vi "Check_Traverse_move.vi"(0 "Current position":dbl[](array[numeric])=[0.0, 0.0, 0.0] format="%.2f", 1 "Traverse Name":string, 2 "Full Check":bool, 5 "New Position":dbl[](array[numeric])=[0.0, 0.0, 0.0] format="%.2f", 7 "Model       Roll      Pitch       Yaw (deg)":dbl[](array[numeric]) format="%#.2f", 9 "Probe Volume":T1=[{"Max"=15.0, "Min"=-15.0}, {"Max"=250.0, "Min"=0.0}, {"Max"=15.0, "Min"=-15.0}] {"Min" format="%#.1f"; "Max" format="%#.1f"}, 11 "Entire Space":T1=[{"Max"=15001.0, "Min"=12000.0}, {"Max"=1000.0, "Min"=-1000.0}, {"Max"=700.0, "Min"=0.0}] {"Min" format="%#.1f"; "Max" format="%#.1f"}, 12 "Exclude Array":T2[](array[typedef])=[{"Sizes"=[{"Max"=15000.0, "Min"=0.0}, {"Max"=1000.0, "Min"=-1000.0}, {"Max"=300.0, "Min"=0.0}], "Name"="Roughness Elements", "Exclude Type"=enum."Allow only vertical moves"}, {"Sizes"=[{"Max"=17000.0, "Min"=16000.0}, {"Max"=200.0, "Min"=-200.0}, {"Max"=-50.0, "Min"=-250.0}], "Name"="B204", "Exclude Type"=enum."Exclude completely"}] {"Sizes"."Min" format="%#.1f"; "Sizes"."Max" format="%#.1f"}, 13 "Probe Support":T1=[{"Max"=15001.0, "Min"=12000.0}, {"Max"=1000.0, "Min"=-1000.0}, {"Max"=700.0, "Min"=0.0}] {"Min" format="%#.1f"; "Max" format="%#.1f"}) -> (6 "Position At Crash":dbl[](array[numeric]) format="%.2f", 10 "Steps":dbl[][](array[numeric]) format="%.2f", 15 "Error Comments":string)   [LabVIEW 2013]
uses:
  Box_size.ctl
  Exclude_cluster.ctl
  Exclusion_type.ctl
panel:
  # "X                Y                   Z"
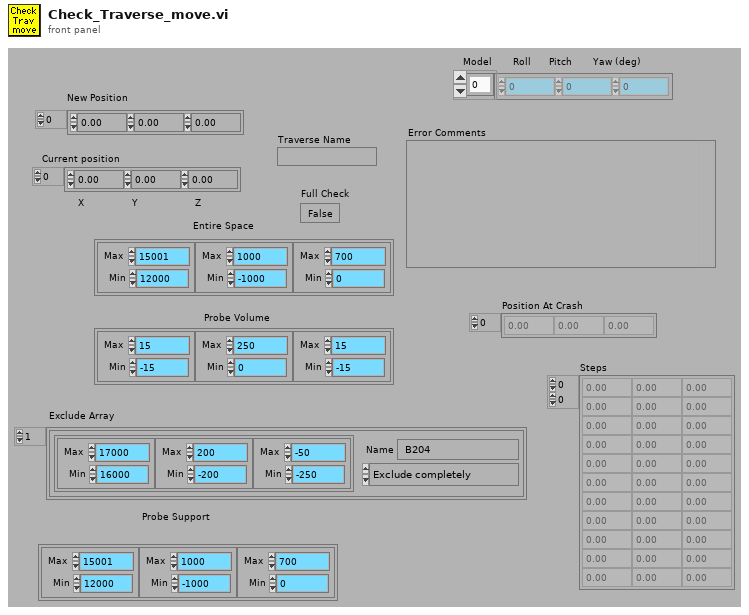
[diagram p1: front panel]
types:
  T1 = typedef "Box_size.ctl" = cluster{"Max":dbl, "Min":dbl}[]
  T2 = typedef "Exclude_cluster.ctl" = cluster{"Sizes":T1, "Name":string, "Exclude Type":T3}
  T3 = typedef "Exclusion_type.ctl" = enum16{"Exclude completely", "Allow only vertical moves"}
  T4 = enum16{"To Traverse Coordinates", "To User Coordinates"}
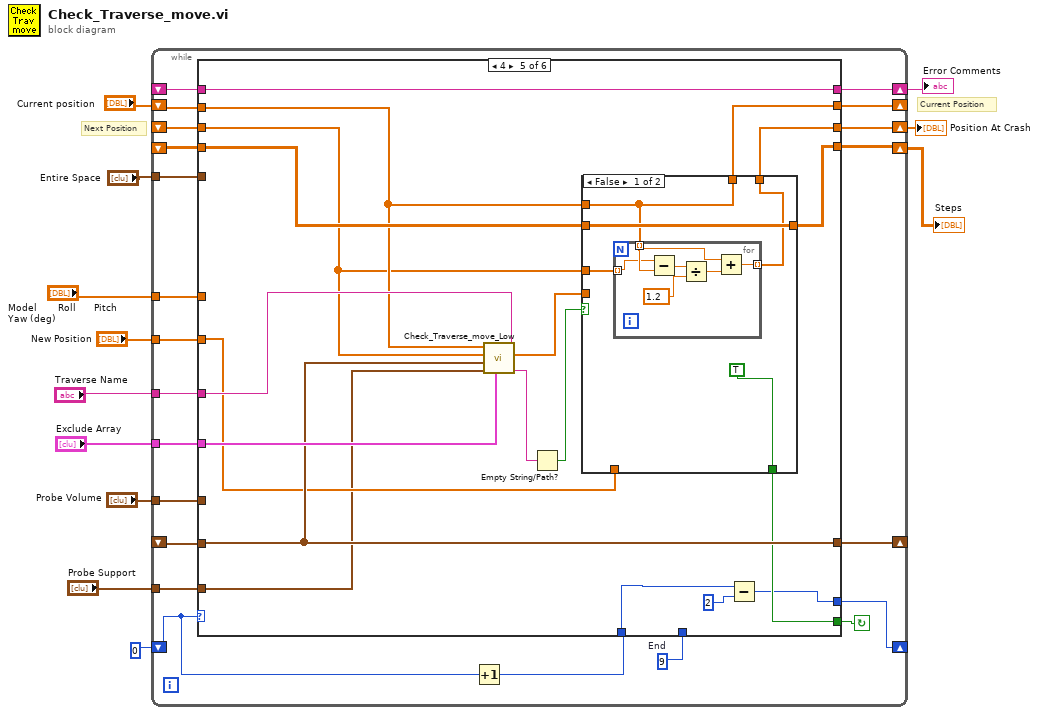
[diagram p0: block diagram]
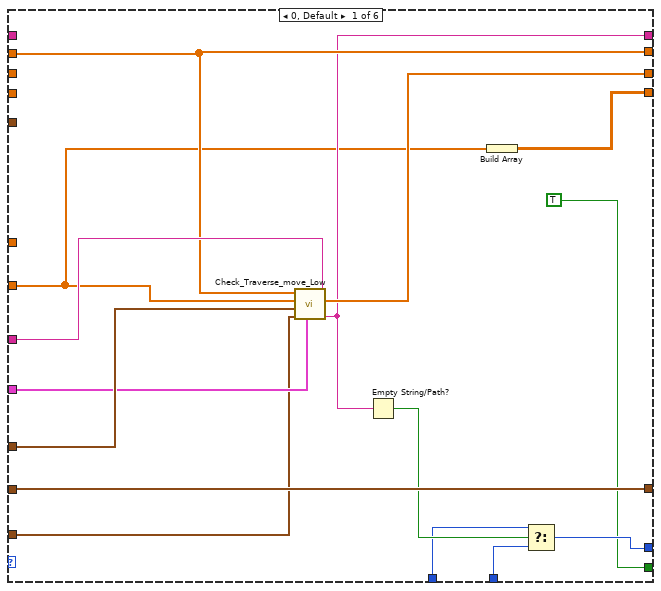
[diagram p2: hidden frame]
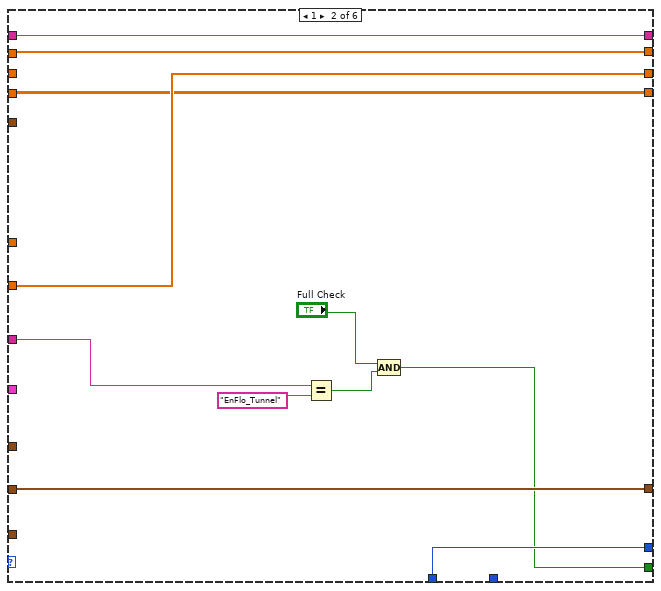
[diagram p3: hidden frame]
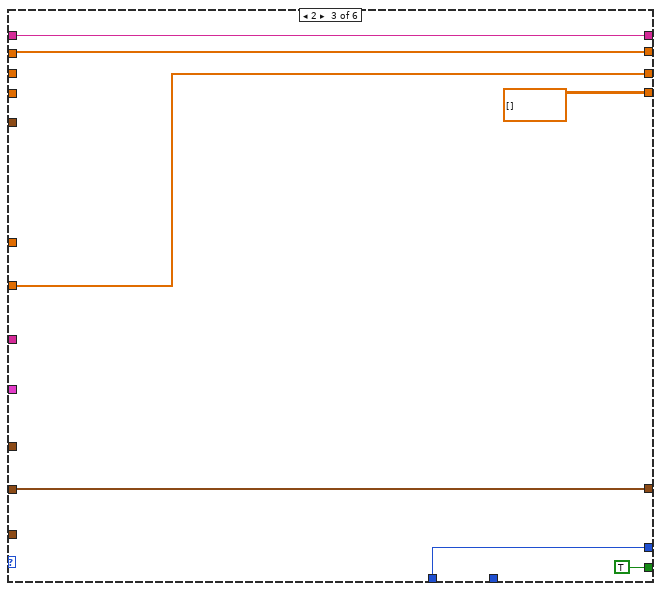
[diagram p4: hidden frame]
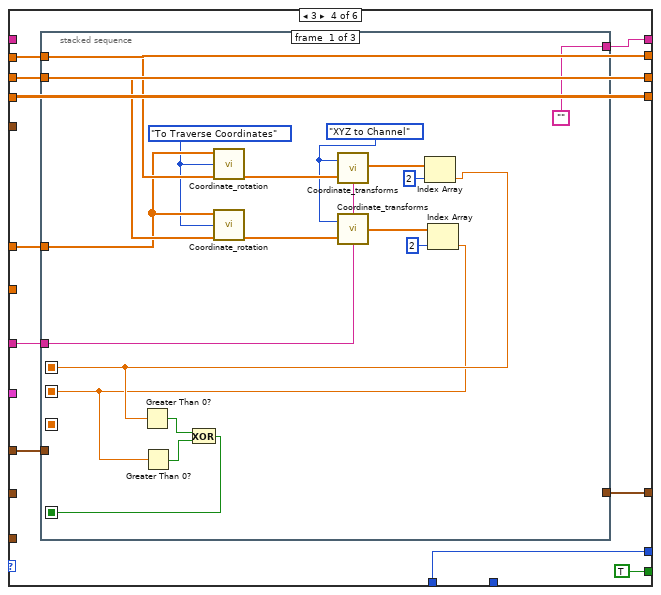
[diagram p5: hidden frame]
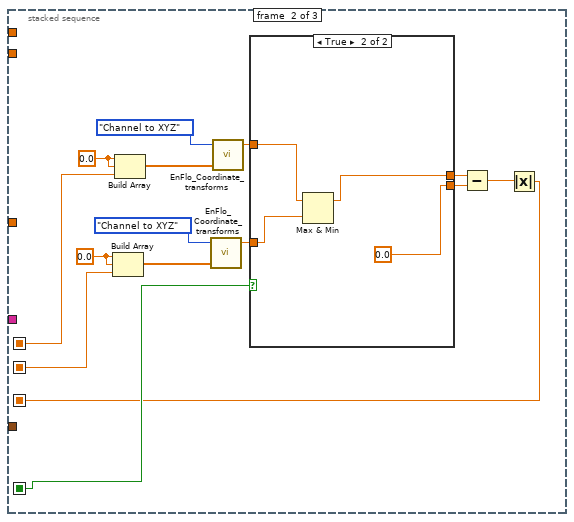
[diagram p6: hidden frame]
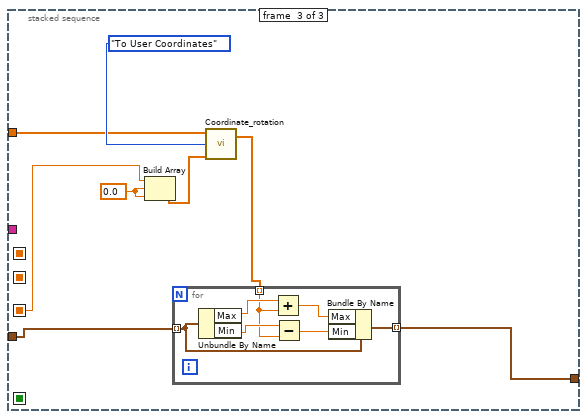
[diagram p8: hidden frame]
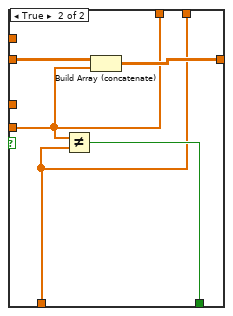
[diagram p9: hidden frame]
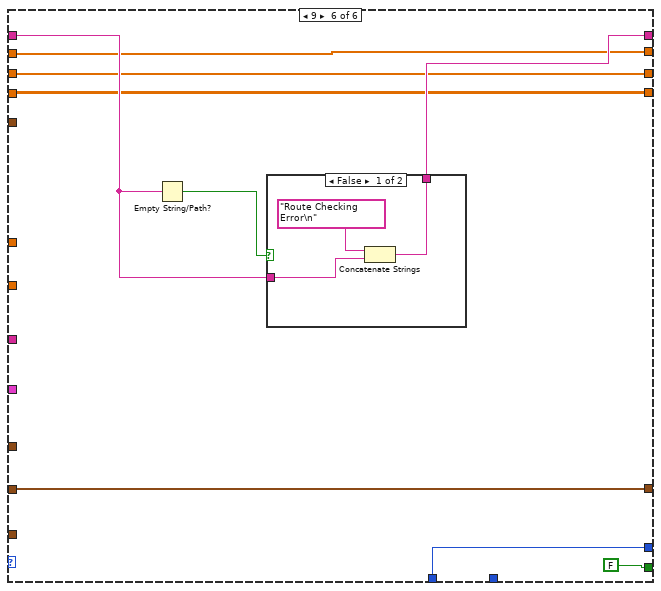
[diagram p10: hidden frame]
diagram:
  # "Current Position"
  # "Next Position"
  n1 = while {
    shift-left: _ -> [w15]
    shift-right: [w14] -> w3
    tunnel: "Probe Volume" -> [w17]
    shift-left: _ -> [w19]
    shift-right: [w18] -> _
    tunnel: "Model       Roll      Pitch       Yaw (deg)" -> [w20]
    tunnel: "New Position" -> [w21]
    shift-left: _ -> [w23]
    shift-right: [w24] -> w7
    shift-left: 0 -> [w27]
    shift-right: [w26] -> _
    tunnel: "Traverse Name" -> [w28]
    tunnel: "Entire Space" -> [w29]
    tunnel: "Exclude Array" -> [w30]
    shift-left: _ -> [w22]
    shift-right: [w32] -> w5
    shift-left: "Current position" -> [w34]
    shift-right: [w33] -> _
    tunnel: "Probe Support" -> [w13]
    stop <- w31 continue-if-true
    w16 = 9  # End
    n2 = Increment(x=w27) -> (x+1=w25:i32)
    n3 = case shown="4" w27 {
      tunnel: w34 -> [w44 w59 w66 w74 w134 w169]
      tunnel: [w44 w59 w66 w74 w139 w169] -> w33
      tunnel: [w47 w52 w63 w73 w138 w168] -> w32
      tunnel: [TRUE ("Box Inside") w54 TRUE ("Box Inside") TRUE ("Box Inside") w141 FALSE ("Box Inside")] -> w31
      tunnel: w19 -> [w46 w58 w65 _ w148 w170]
      tunnel: w30 -> [w48 _ _ _ w150 _]
      tunnel: w29 -> [_ _ _ _ _ _]
      tunnel: w28 -> [w45 w55 _ w71 w149 _]
      tunnel: [w39 w57 w64 w69 w136 w172] -> w26
      tunnel: w25 -> [w41 w57 w64 w69 w135 w172]
      tunnel: [w43 w60 w67 w77 w146 w173] -> w24
      tunnel: w23 -> [_ w60 w67 _ w146 w174]
      tunnel: w22 -> [_ _ _ w73 w133 w168]
      tunnel: w21 -> [w38 w52 w63 _ w142 _]
      tunnel: w20 -> [_ _ _ w72 _ _]
      tunnel: [w46 w58 w65 w75 w148 w170] -> w18
      tunnel: w17 -> [w49 _ _ w70 _ _]
      tunnel: w16 -> [w40 _ _ _ _ _]
      tunnel: w15 -> [_ w51 _ w68 w145 w167]
      tunnel: [w37 w51 dbl[][] [] w68 w144 w167] -> w14
      tunnel: w13 -> [w35 _ _ _ w132 _]
      frame 0, Default {
        n4 = call "Check_Traverse_move_Low.vi"("Traverse Name"=w45, "Exclude Array"=w48, "Probe Support"=w35, "Probe Volume"=w49, "New Position"=w38, "Current position"=w44) -> ("Error Comments"=w43:string, "Position At Crash"=w47:dbl[])  [unwired: 1 in, 1 out]
        n5 = Empty String/Path?(string/path=w43) -> (empty?=w42:bool)
        n6 = Build Array(w38) -> (w37:dbl[][])
        n7 = Select(t=w41, s=w42, f=w40) -> (s? t:f=w39:i32)
      }
      frame 1 {
        n8 = Equal?(x=w55, y="EnFlo_Tunnel") -> (x = y?=w50:bool)
        n9 = Compound Arithmetic op=AND("Full Check", w50) -> (w54:bool)
      }
      frame 2 {
      }
      frame 3 {
        n10 = stacked-sequence {
          seq-local: [w80 _ _] -> [_ w110 _]
          seq-local: [w79 _ _] -> [_ w109 _]
          seq-local: [w78 _ _] -> [_ w100 _]
          seq-local: [_ w96 _] -> [_ _ w119]
          tunnel: ["" _ _] -> w77
          tunnel: [_ _ w123] -> w75
          tunnel: w74 -> [w93 _ _]
          tunnel: w73 -> [w91 _ _]
          tunnel: w72 -> [w90 _ w117]
          tunnel: w71 -> [w89 _ _]
          tunnel: w70 -> [_ _ w124]
          frame #0 {
            w87 = enum16{"XYZ to Channel", "Channel to XYZ"}."XYZ to Channel" ("Mode")
            w88 = T4."To Traverse Coordinates" ("Mode")
            n11 = call "Coordinate_rotation.vi"("Model       Roll      Pitch       Yaw (deg)"=w90, "Input Position"=w93, "Mode"=w88) -> ("Output Position"=w94:dbl[])  [unwired: 2 in, 1 out]
            n12 = call "Coordinate_rotation.vi"("Model       Roll      Pitch       Yaw (deg)"=w90, "Input Position"=w91, "Mode"=w88) -> ("Output Position"=w92:dbl[])  [unwired: 2 in, 1 out]
            n13 = call "Coordinate_transforms.vi"("Traverse Name"=w89, "Input"=w94, "Mode"=w87) -> ("Output"=w86:dbl[])
            n14 = call "Coordinate_transforms.vi"("Traverse Name"=w89, "Input"=w92, "Mode"=w87) -> ("Output"=w83:dbl[])
            n15 = Index Array(array=w86, index=2) -> (element=w80:dbl)
            n16 = Greater Than 0?(x=w80) -> (x > 0?=w82:bool)
            n17 = Index Array(array=w83, index=2) -> (element=w79:dbl)
            n18 = Greater Than 0?(x=w79) -> (x > 0?=w81:bool)
            n19 = Exclusive Or(1:w81, 2:w82) -> (0:w78:bool)
          }
          frame #1 {
            w103 = 0.0 ("element")
            w108 = 0.0 ("element")
            n20 = Build Array(w103, w103, w109) -> (w105:dbl[])
            n21 = Build Array(w108, w108, w110) -> (w106:dbl[])
            n22 = call "EnFlo_Coordinate_transforms.vi"("Input"=w105, "Mode"=enum16{"XYZ to Channel", "Channel to XYZ"}."Channel to XYZ") -> ("X theta"=w101:dbl)  [unwired: 3 out]
            n23 = call "EnFlo_Coordinate_transforms.vi"("Input"=w106, "Mode"=enum16{"XYZ to Channel", "Channel to XYZ"}."Channel to XYZ") -> ("X theta"=w102:dbl)  [unwired: 3 out]
            n24 = case shown="True" w100 {
              tunnel: w102 -> [w112 w115]
              tunnel: w101 -> [w111 w116]
              tunnel: [w111 0.0 ("element")] -> w99
              tunnel: [w112 w114] -> w98
              frame False {
              }
              frame True {
                n25 = Max & Min(x=w115, y=w116) -> (max(x,y)=w114:dbl)  [unwired: 1 out]
              }
            }
            n26 = Subtract(x=w98, y=w99) -> (x-y=w97:dbl)
            n27 = Absolute Value(x=w97) -> (abs(x)=w96:dbl)
          }
          frame #2 {
            w121 = 0.0 ("Input Element")
            n28 = Build Array(w119, w121, w121) -> (w120:dbl[])
            n29 = call "Coordinate_rotation.vi"("Model       Roll      Pitch       Yaw (deg)"=w117, "Input Position"=w120, "Mode"=T4."To User Coordinates") -> ("Output Position"=w118:dbl[])  [unwired: 2 in, 1 out]
            n30 = for {
              tunnel: w124 -> [w131] mode=indexing
              tunnel: w118 -> [w126] mode=indexing
              tunnel: [w125] -> w123 mode=indexing
              n31 = Unbundle By Name(w131) -> ("Max"=w130:dbl, "Min"=w129:dbl)
              n32 = Add(x=w130, y=w126) -> (x+y=w128:dbl)
              n33 = Subtract(x=w129, y=w126) -> (x-y=w127:dbl)
              n34 = Bundle By Name(cluster=w131, "Max"=w128, "Min"=w127) -> (w125:cluster{"Max":dbl, "Min":dbl})
            }
          }
        }
      }
      frame 4 {
        n35 = call "Check_Traverse_move_Low.vi"("Traverse Name"=w149, "Exclude Array"=w150, "Probe Support"=w132, "Probe Volume"=w148, "New Position"=w133, "Current position"=w134) -> ("Error Comments"=w147:string, "Position At Crash"=w140:dbl[])  [unwired: 1 in, 1 out]
        n36 = Empty String/Path?(string/path=w147) -> (empty?=w143:bool)
        n37 = case shown="False" w143 {
          tunnel: w145 -> [w155 w166]
          tunnel: w140 -> [_ w163]
          tunnel: [w155 w165] -> w144
          tunnel: w142 -> [_ w162]
          tunnel: [TRUE w164] -> w141
          tunnel: [w153 w163] -> w139
          tunnel: [w151 w162] -> w138
          tunnel: w134 -> [w153 _]
          tunnel: w133 -> [w152 _]
          frame False {
            n38 = for {
              tunnel: w153 -> [w157] mode=indexing
              tunnel: w152 -> [w156] mode=indexing
              tunnel: [w158] -> w151 mode=indexing
              n39 = Subtract(x=w156, y=w157) -> (x-y=w161:dbl)
              n40 = Divide(x=w161, y=1.2) -> (x/y=w159:dbl)
              n41 = Add(x=w157, y=w159) -> (x+y=w158:dbl)
            }
          }
          frame True {
            n42 = Not Equal?(x=w163, y=w162) -> (x != y?=w164:bool)
            n43 = Build Array (concatenate)(w166, w163) -> (w165:dbl[][])
          }
        }
        n44 = Subtract(x=w135, y=2) -> (x-y=w136:i32)
      }
      frame 9 {
        n45 = Empty String/Path?(string/path=w174) -> (empty?=w175:bool)
        n46 = case shown="False" w175 {
          tunnel: [w176 w179] -> w173
          tunnel: w174 -> [w178 w179]
          frame False {
            n47 = Concatenate Strings("Route Checking Error\n" ("String to match"), w178) -> (w176:string)
          }
          frame True {
          }
        }
      }
    }
  }
  "Error Comments" <- w7
  "Position At Crash" <- w5
  "Steps" <- w3
